vi "test_TxUDP-RxUDP - Multiple Boards - GenXML.vi"(8 "error in":errorcluster, 11 "reference in":refnum<class "AIM ARINC 664 Loopback-MultiDevice.lvclass">) -> (0 "error out":errorcluster, 3 "reference out":refnum<class "AIM ARINC 664 Loopback-MultiDevice.lvclass">)   [LabVIEW 2020, in "AIM ARINC 664 Loopback-MultiDevice.lvclass"]
uses:
  AIM ARINC 664 Loopback-MultiDevice.lvclass
  C:/Program Files/National Instruments/LabVIEW 2024/vi.lib/NI/VeriStand Custom Device Testing Tools/VeriStandTestCase/VeriStandTestCase.lvclass
  AIM ARINC 664 Loopback-MultiDevice.lvclass/AIM ARINC 664 Loopback-MultiDevice.ctl
  b47c41b5-a02e-49d5-b852-4e28f097d7ad.vi
  6a3dd3ed-914d-4d14-bf18-724521aa5e28.vi
  8abe1e9f-12f7-4d29-bb0e-ea5e1950c3f4.vi
  NationalInstruments.VeriStand.SystemDefinitionAPI
  <vilib>/addons/_JKI Toolkits/VI Tester/TestCase.llb/TestCase.lvclass
  Scripting/AIM ARINC 664 Scripting.lvlib
  Import/AIM ARINC 664 Import.lvlib
  <vilib>/NI/VeriStand Custom Device Testing Tools/VeriStandTestCase/VeriStandTestCase.lvclass
  C:/Program Files/National Instruments/LabVIEW 2024/vi.lib/addons/_JKI Toolkits/VI Tester/TestCase.llb/TestCase.lvclass
panel:
  out "resulting string":string
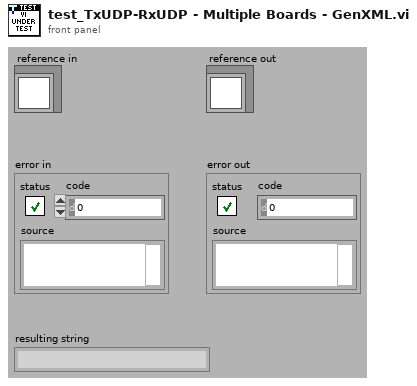
[diagram p1: front panel]
types:
  T1 = typedef "Custom Device API.lvlib/Custom Device Item Ref.ctl" = u64
  T2 = typedef "AIM ARINC 664 Import.lvlib/Board Top Level Configuration.ctl" = cluster{"boardSetup":T3, "portConfiguration":T4[]}
  T3 = typedef "AIM ARINC 664 Import.lvlib/board_setup.ctl" = cluster{"boardId":u32, "portSpeed":u32, "portConfig":u32}
  T4 = typedef "AIM ARINC 664 Import.lvlib/port_configuration.ctl" = cluster{"portSetup":T5, "Tx_Generic":T6[], "Rx_Monitor":cluster{"DefaultCronoMode":u32, "GlbMonBufferSizeIn":u32, "CaptureMode":u32, "MaxFileSizeMB":u32, "Strobe":u32, "TriggerPosition":u32}[], "Tx_UDP":cluster{"tx_udp_setup":cluster{"VlId":i32, "Bag":i32, "NetSelect":u32, "domainID":u8, "sideID":u8, "locationID":u8, "interfaceID":u8, "NumOfSubVl":u16, "Skew":u32, "MaxFrameLength":u32, "FrameBufferSize":u32}, "commPorts":T14[], "sapPorts":T15[]}[], "Rx_UDP":cluster{"Tx_UDP":T16, "commPorts":T17[], "sapPorts":T18[]}[]}
  T5 = typedef "AIM ARINC 664 Import.lvlib/port_setup.ctl" = cluster{"port Id":u32, "redundant":bool}
  T6 = typedef "AIM ARINC 664 Import.lvlib/session_tx_generic.ctl" = cluster{"tx_generic_setup":T7, "Frame Headers":T8[]}
  T7 = typedef "AIM ARINC 664 Import.lvlib/tx_generic_setup.ctl" = cluster{"QueueSizeIn":u32, "Count":i32, "StartMode":i32}
  T8 = typedef "AIM ARINC 664 Import.lvlib/frame_tx_generic.ctl" = cluster{"FrameID":string, "PayloadID":string, "Frame header":cluster{"FrameStartMode":i32, "InterFrameGap":i32, "PacketGroupWaitTime":i32, "NetSelect":u32, "PayloadBufferMode":i32, "PayloadGenerationMode":i32, "PhysErrorInjection":i32, "PreambleCount":i32, "SequenceNumberInit":T9, "SequenceNumberOffset":T10, "Skew":i32}, "Parameters":T11[]}
  T9 = typedef "AIM ARINC 664 Import.lvlib/frame_tx_generic_seqNumberInit.ctl" = i32
  T10 = typedef "AIM ARINC 664 Import.lvlib/frame_tx_generic_seqNumberOffset.ctl" = i32
  T11 = typedef "AIM ARINC 664 Import.lvlib/frame_parameter.ctl" = cluster{"name":string, "default value":dbl, "unit":string, "Parameter":T12}
  T12 = typedef "AIM ARINC 664 Import.lvlib/frame_parameter_definition.ctl" = cluster{"start index":i32, "size":i32, "encoding":T13, "signed":bool, "scale multiplier":dbl, "scale offset":dbl}
  T13 = typedef "Encoding (Arinc664).ctl" = u16
  T14 = typedef "AIM ARINC 664 Import.lvlib/port_tx_udp_comm.ctl" = cluster{"PayloadID":string, "partitionID":u8, "UdpSrcPort":u16, "UdpDstPort":u16, "PortType":enum16{"FDX_UDP_SAMPLING", "FDX_UDP_QUEUING"}, "SubVIId":u32, "UdpNumBufMessages":u32, "UdpMaxMessageSize":u32, "UdpSamplingRate":u32, "Parameters":T11[]}
  T15 = typedef "AIM ARINC 664 Import.lvlib/port_tx_udp_sap.ctl" = cluster{"PayloadID":string, "SubVlId":u8, "UdpSrcPort":u16, "UdpNumBufMessages":u32, "UdpMaxMessageSize":u32, "partitionID":u8, "domainID":u8, "sideID":u8, "locationID":u8, "interfaceID":u8, "Parameters":T11[]}
  T16 = typedef "AIM ARINC 664 Import.lvlib/rx_udp_setup.ctl" = cluster{"VerificationMode":u32, "Bag":u32, "Jitter":u32, "MaxFrameLength":u32, "MaxSkew":u32, "VLBufSize":u32, "FilterMode":u32, "FilterPosition":u32, "Padding":u32, "FilterMask":u32, "FilterData":u32, "MinFrameLength":u32, "VlId":u16, "VLRange":u32}
  T17 = typedef "AIM ARINC 664 Import.lvlib/port_rx_udp_comm.ctl" = cluster{"PayloadID":string, "domainID":u8, "sideID":u8, "locationID":u8, "partitionID":u8, "UdpSrcPort":u16, "UdpDstPort":u16, "PortType":enum16{"FDX_UDP_SAMPLING", "FDX_UDP_QUEUING"}, "SubVIId":u32, "UdpNumBufMessages":u32, "UdpMaxMessageSize":u32, "UdpSamplingRate":u32, "Parameters":T11[]}
  T18 = typedef "AIM ARINC 664 Import.lvlib/port_rx_udp_sap.ctl" = cluster{"PayloadID":string, "UdpDstPort":u16, "UdpNumBufMessages":u32, "UdpMaxMessageSize":u32, "Parameters":T11[]}
  T19 = typedef "Payload Map.ctl" = map{string, T20}
  T20 = typedef "Payload Record Type.ctl" = cluster{"Data":u8[], "Type of Frame":T21}
  T21 = typedef "Type of Payload.ctl" = u16
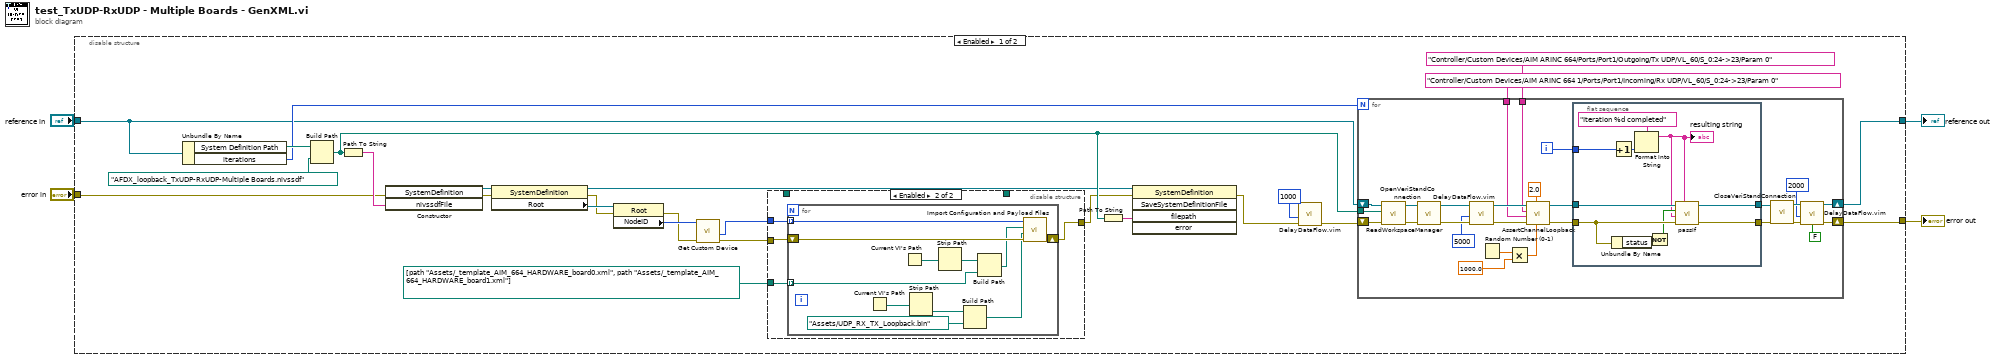
[diagram p0: block diagram]
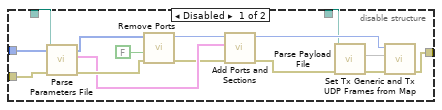
[diagram p2: hidden frame]
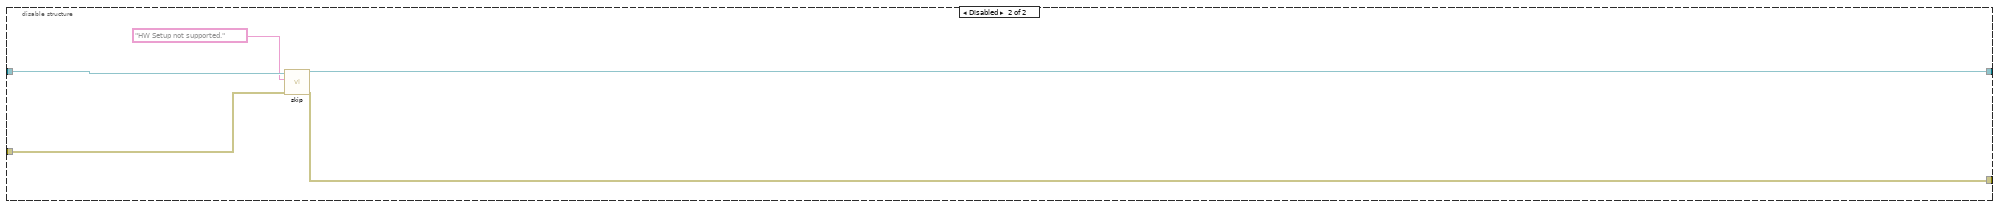
[diagram p3: hidden frame]
diagram:
  n1 = disable-structure shown="Enabled" {
    disable-tunnel: "reference in" -> [w8 w99]
    disable-tunnel: "error in" -> [w7 w98]
    disable-tunnel: [w28 w97] -> w2
    disable-tunnel: [w27 w96] -> w1
    frame Enabled {
      n2 = Unbundle By Name(w8) -> ("System Definition Path"=w30:path, "iterations"=w14:i32)
      n3 = Build Path(base path=w30, name or relative path=path "AFDX_loopback_TxUDP-RxUDP-Multiple Boards.nivssdf") -> (appended path=w25:path)
      n4 = Path To String(path=w25) -> (string=w26:string)
      n5 = constructor class="SystemDefinition"(error in=w7, "nivssdfFile"=w26) -> (reference out=w24:refnum<k24>, error out=w22:errorcluster)  [unwired: 2 in, 2 out]
      n6 = property class="SystemDefinition"(reference=w24, error in=w22) -> (reference out=w19:refnum<k24>, error out=w21:errorcluster, "Root"=w23:refnum<k24>)
      n7 = property class="Root"(reference=w23, error in=w21) -> (error out=w16:errorcluster, "NodeID"=w17:u64)  [unwired: 1 out]
      n8 = call "Get Custom Device.vi"("error in"=w16, "custom device ref in"=w17) -> ("error out"=w15:errorcluster, "Item Refs"=w6:T1[])  [unwired: 5 in, 3 out]
      n9 = disable-structure shown="Enabled" {
        disable-tunnel: w6 -> [w78 w82]
        disable-tunnel: w15 -> [w70 w83]
        disable-tunnel: _ -> [w68 _]
        disable-tunnel: _ -> [w67 _]
        disable-tunnel: [w66 w81] -> w20
        disable-tunnel: path[] [path "Assets/_template_AIM_664_HARDWARE_board0.xml", path "Assets/_template_AIM_664_HARDWARE_board1.xml"] -> [_ w80]
        frame Disabled {
          n10 = call "Parse Parameters File.vi"("error in"=w70, "path to XML document"=w67) -> ("error out"=w79:errorcluster, "board configuration out"=w76:T2)  [unwired: 7 in, 1 out]
          n11 = call "Remove Ports.vi"("error in"=w79, "refresh?"=FALSE, "Custom device Ref"=w78) -> ("error out"=w75:errorcluster, "Custom device Ref out"=w77:T1)  [unwired: 7 in]
          n12 = call "Add Ports and Sections.vi"("error in"=w75, "board configuration in"=w76, "custom device ref"=w77) -> ("error out"=w74:errorcluster, "custom device ref out"=w69:T1)  [unwired: 7 in]
          n13 = call "Parse Payload File.vi"("error in"=w74, "frame array path in"=w68) -> ("error out"=w73:errorcluster, "Map"=w72:T19)  [unwired: 7 in, 1 out]
          n14 = call "Set Tx Generic and Tx UDP Frames from Map.vi"("error in"=w73, "payload map"=w72, "custom device ref"=w69) -> ("error out"=w66:errorcluster)  [unwired: 7 in, 1 out]
        }
        frame Enabled {
          n15 = for {
            shift-right: [w93] -> w81
            shift-left: w83 -> [w94]
            tunnel: w80 -> [w86] mode=indexing
            tunnel: w82 -> [w85] mode=indexing
            n16 = Current VI's Path() -> (path=w91:path)
            n17 = Current VI's Path() -> (path=w88:path)
            n18 = Strip Path(path=w91) -> (stripped path=w92:path)  [unwired: 1 out]
            n19 = Strip Path(path=w88) -> (stripped path=w89:path)  [unwired: 1 out]
            n20 = Build Path(base path=w92, name or relative path=path "Assets/UDP_RX_TX_Loopback.bin") -> (appended path=w90:path)
            n21 = Build Path(base path=w89, name or relative path=w86) -> (appended path=w87:path)
            n22 = call "Import Configuration and Payload Files.vi"("error in"=w94, "payload file path"=w90, "parameters configuration file path"=w87, "custom device ref"=w85) -> ("error out"=w93:errorcluster)  [unwired: 6 in, 1 out]
          }
        }
      }
      n23 = Path To String(path=w25) -> (string=w18:string)
      n24 = invoke class="SystemDefinition" method="SaveSystemDefinitionFile"(reference=w19, error in=w20, "filepath"=w18) -> (error out=w13:errorcluster)  [unwired: 2 in, 4 out]
      n25 = call "DelayDataFlow.vim"("value in"=w13, "milliseconds to wait"=u32 1000) -> ("value out"=w12:errorcluster)  [unwired: 2 in, 1 out]
      n26 = for {
        N: w14 -> [_]
        tunnel: w25 -> [w48]
        shift-right: [w53] -> w27
        shift-left: w8 -> [w55]
        shift-right: [w43] -> w28
        shift-left: w12 -> [w49]
        tunnel: "Controller/Custom Devices/AIM ARINC 664 1/Ports/Port1/Incoming/Rx UDP/VL_60/S_0:24->23/Param 0" -> [w35]
        tunnel: "Controller/Custom Devices/AIM ARINC 664/Ports/Port1/Outgoing/Tx UDP/VL_60/S_0:24->23/Param 0" -> [w34]
        i -> [w37]
        n27 = call-dynamic "OpenVeriStandConnection.vi"("error in (no error)"=w49, "System Definition File"=w48, "VeriStand Test Case in"=w55) -> ("error out"=w54:errorcluster, "VeriStand Test Case out"=w52:refnum<class "AIM ARINC 664 Loopback-MultiDevice.lvclass">)  [unwired: 6 in, 1 out]
        n28 = call-dynamic "ReadWorkspaceManager.vi"("error in (no error)"=w54, "VeriStand Test Case in"=w52) -> ("error out"=w51:errorcluster, "VeriStand Test Case out"=w46:refnum<class "AIM ARINC 664 Loopback-MultiDevice.lvclass">)  [unwired: 7 in, 1 out]
        n29 = call "DelayDataFlow.vim"("value in"=w51, "milliseconds to wait"=u32 5000) -> ("value out"=w47:errorcluster)  [unwired: 2 in, 1 out]
        n30 = Random Number (0-1)() -> (number: 0 to 1=w33:dbl)
        n31 = Multiply(x=w33, y=1000.0 ("Value")) -> (x*y=w31:dbl)
        n32 = call <vilib>:"AssertChannelLoopback.vi"("Value"=w31, "Timeout (1 second)"=2.0, "error in (no error)"=w47, "Read Channel"=w35, "Write Channel"=w34, "VeriStand Test Case in"=w46) -> ("error out"=w38:errorcluster, "VeriStand Test Case out"=w36:refnum<class "AIM ARINC 664 Loopback-MultiDevice.lvclass">)  [unwired: 4 in]
        n33 = flat-sequence {
          tunnel: [w65] -> w40
          tunnel: [w64] -> w39
          tunnel: w38 -> [w63]
          tunnel: w37 -> [w59]
          tunnel: w36 -> [w57]
          frame #0 {
            n34 = Unbundle By Name(w63) -> ("status"=w62:bool)
            n35 = Increment(x=w59) -> (x+1=w58:i32)
            n36 = Format Into String(format string="Iteration %d completed", w58) -> (resulting string=w56:string)  [unwired: 2 in, 1 out]
            "resulting string" <- w56
            n37 = Not(x=w62) -> (.not. x?=w61:bool)
            n38 = call-dynamic "passIf.vi"("custom report message (\"\")"=w56, "error in (no error)"=w63, "message (\"\")"=w56, "pass"=w61, "TestCase in"=w57) -> ("error out"=w64:errorcluster, "TestCase out"=w65:refnum<class "AIM ARINC 664 Loopback-MultiDevice.lvclass">)  [unwired: 5 in]
          }
        }
        n39 = call-dynamic "CloseVeriStandConnection.vi"("error in (no error)"=w39, "VeriStand Test Case in"=w40) -> ("error out"=w44:errorcluster, "VeriStand Test Case out"=w53:refnum<class "AIM ARINC 664 Loopback-MultiDevice.lvclass">)  [unwired: 8 in]
        n40 = call "DelayDataFlow.vim"("value in"=w44, "milliseconds to wait"=u32 2000, "no delay on error (T)"=FALSE) -> ("value out"=w43:errorcluster)  [unwired: 1 in, 1 out]
      }
    }
    frame Disabled {
      n41 = call <vilib>:"skip.vi"("error in (no error)"=w98, "skipMessage"="HW Setup not supported.", "TestCase in"=w99) -> ("error out"=w97:errorcluster, "TestCase out"=w96:refnum<class "AIM ARINC 664 Loopback-MultiDevice.lvclass">)  [unwired: 7 in]
    }
  }
  "error out" <- w2
  "reference out" <- w1
